vi "Set Temperature.vi"(8 "error in (no error)":errorcluster, 11 "Cooler in":refnum<class "Simulated_Cooler.lvclass">) -> (0 "error out":errorcluster, 3 "Cooler out":refnum<class "Simulated_Cooler.lvclass">)   [LabVIEW 2018, in "Simulated_Cooler.lvclass"]
uses:
  Simulated_Cooler.lvclass
  Simulated_Cooler.lvclass/Simulated_Cooler.ctl
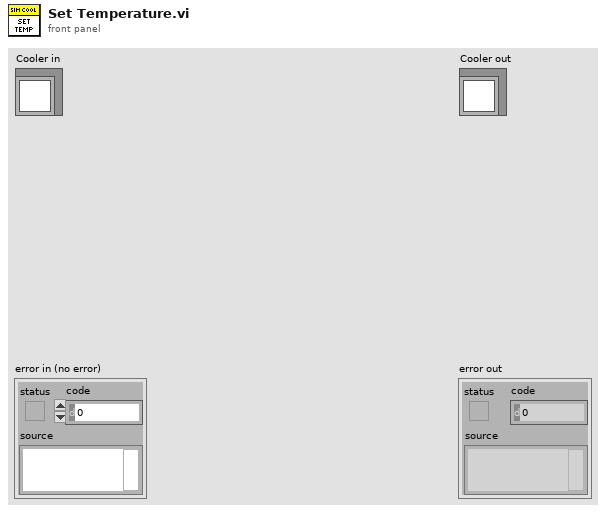
[diagram p1: front panel]
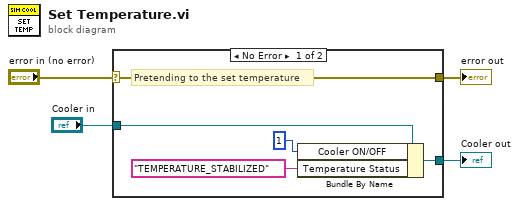
[diagram p0: block diagram]
diagram:
  n1 = case shown="No Error" "error in (no error)" {
    selector: "error in (no error)" -> [w9 w11]
    tunnel: [w9 w11] -> w2
    tunnel: [w6 w10] -> w3
    tunnel: "Cooler in" -> [w7 w10]
    frame No Error {
      # "Pretending to the set temperature"
      n2 = Bundle By Name(cluster=w7, "Cooler ON/OFF"=u8 1, "Temperature Status"="TEMPERATURE_STABILIZED") -> (w6:refnum<class "Simulated_Cooler.lvclass">)
    }
    frame Error {
    }
  }
  "error out" <- w2
  "Cooler out" <- w3
